vi "Broadcast.vi"(6 "Timeout ms (1000)":i32=1000, 7 "Format (Text)":T1, 8 "error in (no error)":errorcluster, 10 "Payload":string, 11 "Basic WebSocket Manager in":refnum<class "Basic WebSocket Manager.lvclass">) -> (0 "error out":errorcluster, 3 "Basic WebSocket Manager out":refnum<class "Basic WebSocket Manager.lvclass">)   [LabVIEW 2020, in "HTTP Server.lvlib" / "Basic WebSocket Manager.lvclass"]
uses:
  Basic WebSocket Manager.lvclass
  Basic WebSocket Manager.lvclass/Basic WebSocket Manager.ctl
  WebSocket Client/WebSocket Client.lvclass
  WebSocket Format.ctl
  HTTP Server.lvlib
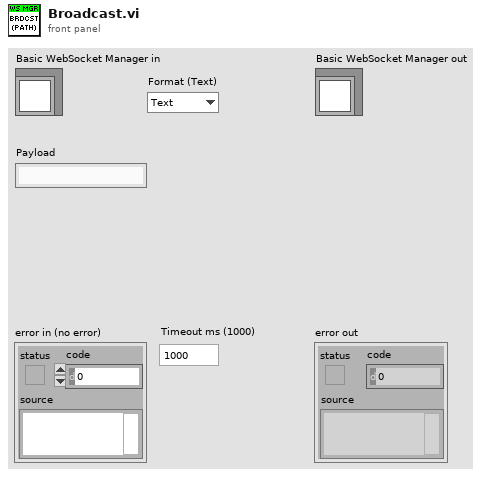
[diagram p1: front panel]
types:
  T1 = typedef "HTTP Server.lvlib/WebSocket Format.ctl" = enum16{"Text", "Binary"}
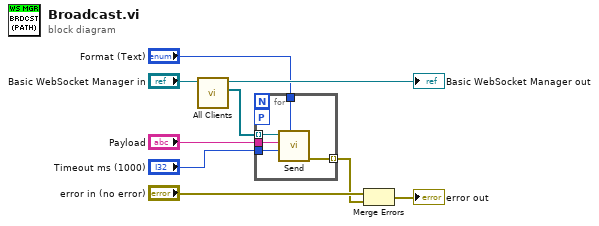
[diagram p0: block diagram]
diagram:
  n1 = call "All Clients.vi"("Basic WebSocket Manager in"="Basic WebSocket Manager in") -> ("Clients"=w6:refnum<class "WebSocket Client.lvclass">[], "Basic WebSocket Manager out"=→"Basic WebSocket Manager out":refnum<class "Basic WebSocket Manager.lvclass">)  [unwired: 8 in, 1 out]
  n2 = for {
    tunnel: w6 -> [w14] mode=indexing
    tunnel: "Payload" -> [w13]
    tunnel: "Timeout ms (1000)" -> [w12]
    tunnel: "Format (Text)" -> [w11]
    tunnel: [w10] -> w1 mode=indexing
    workers-P: _ -> [_]
    n3 = call "Send.vi"("Format (Text)"=w11, "Timeout ms (1000)"=w12, "Payload"=w13, "WebSocket Client in"=w14) -> ("error out"=w10:errorcluster)  [unwired: 6 in, 1 out]
  }
  n4 = Merge Errors("error in (no error)", w1) -> (→"error out":errorcluster)
